vi "FXP_L_ye_Bend_u_singleAxis_32bit.vi"(7 "NS":u8=5, 8 "U(k): ux":fxp<+/-,18,5>, 11 "Y(k): x":fxp<+/-,18,5>) -> (0 "yd_est":fxp<+/-,32,5>, 2 "outputValid":bool, 4 "x0":T1)   [LabVIEW 2017]
uses:
  typeDefs/x_vec_type.ctl
  <vilib>/Platform/TimedLoop/XDataNode/timing_clust.ctl
  <vilib>/Platform/TimedLoop/XDataNode/nitl_modes.ctl
  <vilib>/Platform/TimedLoop/XDataNode/wakeup.ctl
  typeDefs/Lz_bram.ctl
  typeDefs/Bz_bram.ctl
  typeDefs/x_vec_bram.ctl
  <vilib>/rvi/Emulation/niFpgaSctlEmulationGetInTimedLoop.vi
  <vilib>/rvi/Emulation/niFpgaEmulationReportErrorSimple.vi
  <vilib>/rvi/Emulation/niFpgaGetClockAttributes.vi
  <vilib>/rvi/Emulation/niFpgaCriticalErrorInLSC.vi
  <vilib>/rvi/DataTransferAndStorage/Container/Common/niFpgaContainerExecOnDevCompGetState.vi
  <vilib>/rvi/Emulation/niFpgaEmulationIsFPGAContextNoSignature.vi
  <vilib>/rvi/DataTransferAndStorage/Container/Common/niFpgaContainerGetUniqueNameForEmu.vi
  <vilib>/rvi/Emulation/niFpgaProcessEmulError.vi
  <vilib>/rvi/errors/nirviReportUnexpectedCaseInternalError (U32).vi
  <vilib>/rvi/Memory/Memory_Emulation/niFpgaMemoryEmulationCacheClearOnFirstRun.vi
  <vilib>/rvi/Memory/Memory_Emulation/nirvimemoryEmulationManagerCache_MakeExclusive.vi
  <vilib>/rvi/Memory/Memory_Emulation/niFpgaMemoryEmulationValidateCache.vi
  <vilib>/rvi/Memory/Memory_Emulation/nirvimemoryEmulationManagerCache_InsertValue.vi
  <vilib>/Utility/error.llb/Clear Errors.vi
  <vilib>/rvi/Memory/Memory_Emulation/nirvimemoryEmulationManagerCache_ReleaseExclusive.vi
  <vilib>/rvi/Memory/Memory_Emulation/nirvimemoryEmulationManagerCache_GetValue.vi
  <vilib>/rvi/Memory/Memory_Emulation/nirvimemoryEmulationManagerCache_SetValue.vi
  <vilib>/rvi/Emulation/niFpgaSctlEmulationResourceMgr.vi
  <vilib>/Platform/TimedLoop/XDataNode/XDataNode.xnode
  <vilib>/rvi/DataTransferAndStorage/Container/XNode/niFpgaContainer.xnode
  <vilib>/rvi/Memory/Memory_Emulation/niFpgaMemoryEmulationRefIn.vi
  <vilib>/rvi/FXPMathLib/FxpAdd/XNode/nifxpmath_Add.xnode
  <vilib>/Platform/TimedLoop/XDataNode/XDNodeRunTimeDep.lvlib
  <vilib>/rvi/FXPMathLib/sim/FxpSim.dll
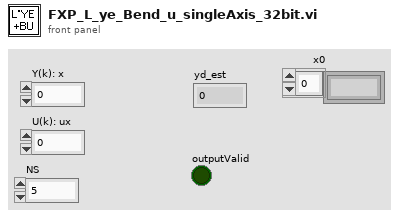
[diagram p1: front panel]
types:
  T1 = typedef "x_vec_type.ctl" = fxp<+/-,32,6>[]
  T2 = typedef "XDNodeRunTimeDep.lvlib/timing_clust.ctl" = cluster{"Expected End [f-1]":u64, "Actual End [f-1]":u64, "Finished Late? [f-1]":bool, "Expected End [i-1]":u64, "Actual End [i-1]":u64, "Finished Late? [i-1]":bool, "Expected Start [i]":u64, "Actual Start [i]":u64, "Expected Start [f]":u64, "Actual Start [f]":u64, "Source Name":string, "Structure Name":string, "Period":i64, "Deadline":i64, "Offset":i64, "Start":i64, "Priority":i32, "Timeout":i32, "Mode":T3, "Wakeup Reason":T4, "Error":errorcluster, "Source Type":string, "Secondary Source Type":string, "Global End Time":u64, "Global Start Time":u64, "Frame Duration":u64, "Iteration Duration":u64, "Assigned CPU":i32, "I/O Scan Engine Mode":u32}
  T3 = typedef "XDNodeRunTimeDep.lvlib/nitl_modes.ctl" = enum32{"No Change", "Process missed periods, maintain original phase", "Discard missed periods, maintain original phase", "Process missed periods, ignore original phase", "Discard missed periods, ignore original phase"}
  T4 = typedef "XDNodeRunTimeDep.lvlib/wakeup.ctl" = enum32{"Normal", "Aborted", "Asynchronous wakeup", "Timing source error", "Timed loop error", "Timeout"}
  T5 = typedef "x_vec_bram.ctl" = refnum<k21>
  T6 = typedef "Bz_bram.ctl" = refnum<k21>
  T7 = typedef "Lz_bram.ctl" = refnum<k21>
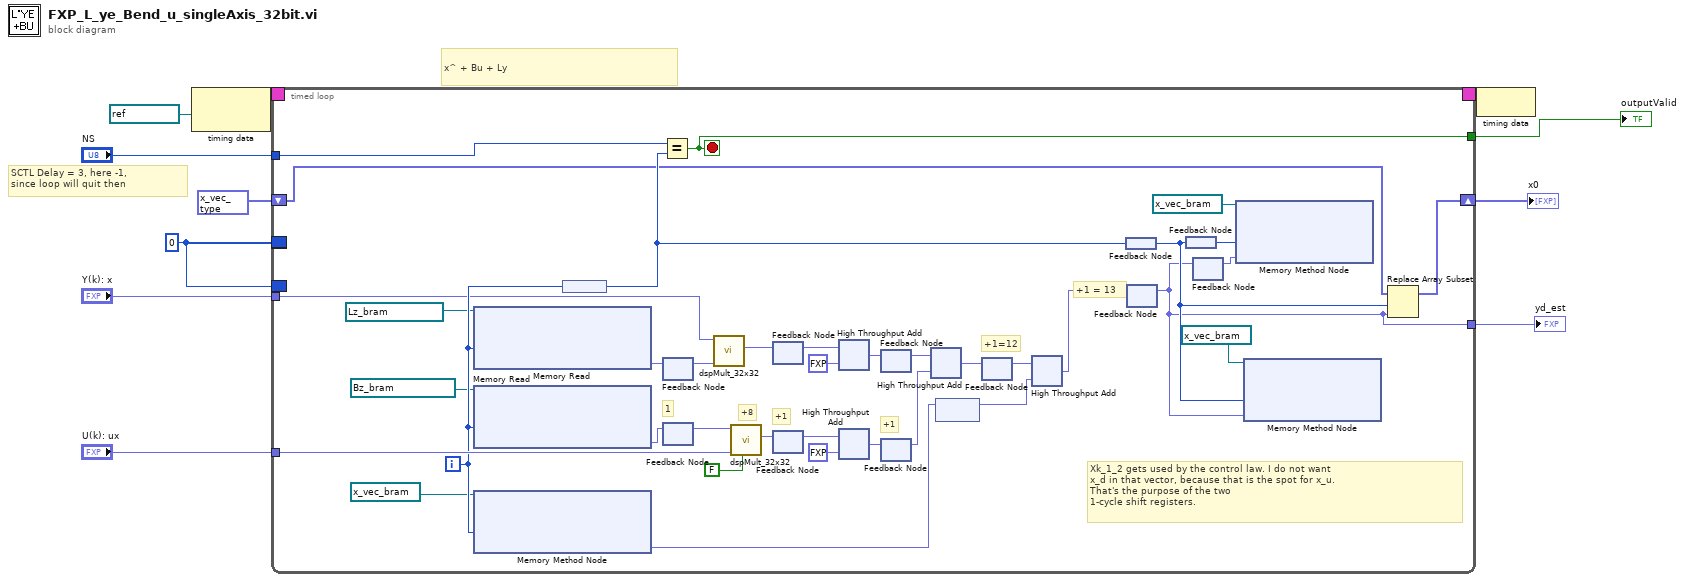
[diagram p0: block diagram]
diagram:
  w6 = 0
  # "x^ + Bu + Ly"
  # "SCTL Delay = 3, here -1,\nsince loop will quit then"
  n1 = node-c288(refnum<k21> "80MHz" ("Source Name")) -> (w11:T2)
  n2 = timed-loop {
    timing: w11 -> [_]
    timing-out: [_] -> w10
    tunnel: "NS" -> [w48]
    border: w6 -> [_]
    tunnel: [w46] -> w8
    border: w6 -> [_]
    tunnel: "Y(k): x" -> [w23]
    tunnel: "U(k): ux" -> [w28]
    border: w6 -> [_]
    tunnel: [w17] -> w5
    shift-right: [w20] -> w2
    shift-left: T1 [0.0, 0.0, 0.0, 0.0, 0.0, 0.0, 0.0, 0.0, 0.0, 0.0, 0.0, 0.0, 0.0, 0.0, 0.0, 0.0, 0.0, 0.0, 0.0, 0.0, 0.0, 0.0, 0.0, 0.0, 0.0] ("Array") -> [w19]
    i -> [w26]
    stop <- w46 stop-if-true
    # "+1 = 13"
    # "+1=12"
    # "+1"
    # "+1"
    # "+8"
    # "1"
    # "Xk_1_2 gets used by the control law. I do not want\nx_d in that vector, because that is the spot for x_u.\nThat's the purpose of the two \n1-cycle shift registers."
    n3 = xnode ("Memory Read")("Address"=w26, "Memory In"=T7 "L_FXP_col1" ("Memory")) -> ("Data"=w44:fxp<+/-,32,3>)  [unwired: 1 out]
    n4 = xnode ("Memory Read")("Address"=w26, "Memory In"=T6 "Bz_FXP_col1" ("Memory")) -> ("Data"=w47:fxp<+/-,32,3>)  [unwired: 1 out]
    n5 = xnode ("Memory Method Node")("Address"=w26, "Memory In"=T5 "xk_1_0" ("Memory")) -> ("Data"=w45:fxp<+/-,32,6>)  [unwired: 1 out]
    n6 = feedback #1() -> (w34:i32)
    n7 = feedback-in #1(w26) -> ()
    n8 = Equal?(x=w48, y=w34) -> (x = y?=w46:bool)
    n9 = feedback #2() -> (w31:fxp<+/-,32,3>)  [unwired: 1 in]
    n10 = feedback-in #2(w44) -> ()
    n11 = feedback #3() -> (w30:fxp<+/-,32,3>)  [unwired: 1 in]
    n12 = feedback-in #3(w47) -> ()
    n13 = call "dspMult_32x32.vi"("b"=w31, "a"=w23) -> ("p"=w32:fxp<+/-,64,10>)  [unwired: 9 in]
    n14 = call "dspMult_32x32.vi"("sclr"=FALSE ("input valid"), "b"=w28, "a"=w30) -> ("p"=w29:fxp<+/-,64,10>)  [unwired: 8 in]
    n15 = feedback #4() -> (w41:fxp<+/-,64,10>)  [unwired: 1 in]
    n16 = feedback-in #4(w32) -> ()
    n17 = feedback #5() -> (w38:fxp<+/-,64,10>)  [unwired: 1 in]
    n18 = feedback-in #5(w29) -> ()
    n19 = xnode ("High Throughput Add")("x"=w41, "y"=fxp<+/-,64,10> 0.0) -> ("x+y"=w40:fxp<+/-,32,8>)
    n20 = xnode ("High Throughput Add")("x"=w38, "y"=fxp<+/-,64,10> 0.0) -> ("x+y"=w37:fxp<+/-,32,8>)
    n21 = feedback #6() -> (w39:fxp<+/-,32,8>)  [unwired: 1 in]
    n22 = feedback-in #6(w40) -> ()
    n23 = feedback #7() -> (w36:fxp<+/-,32,8>)  [unwired: 1 in]
    n24 = feedback-in #7(w37) -> ()
    n25 = xnode ("High Throughput Add")("x"=w39, "y"=w36) -> ("x+y"=w43:fxp<+/-,32,8>)
    n26 = feedback #8() -> (w35:fxp<+/-,32,6>)  [unwired: 1 in]
    n27 = feedback-in #8(w45) -> ()
    n28 = feedback #9() -> (w42:fxp<+/-,32,8>)  [unwired: 1 in]
    n29 = feedback-in #9(w43) -> ()
    n30 = xnode ("High Throughput Add")("x"=w42, "y"=w35) -> ("x+y"=w21:fxp<+/-,32,5>)
    n31 = feedback #10() -> (w18:i32)
    n32 = feedback-in #10(w34) -> ()
    n33 = feedback #11() -> (w17:fxp<+/-,32,5>)  [unwired: 1 in]
    n34 = feedback-in #11(w21) -> ()
    n35 = feedback #12() -> (w22:i32)
    n36 = feedback-in #12(w18) -> ()
    n37 = feedback #13() -> (w33:fxp<+/-,32,5>)  [unwired: 1 in]
    n38 = feedback-in #13(w17) -> ()
    n39 = xnode ("Memory Method Node")("Address"=w22, "Data"=w33, "Memory In"=T5 "xk_1_2" ("Memory")) -> ()  [unwired: 1 out]
    n40 = xnode ("Memory Method Node")("Address"=w18, "Data"=w17, "Memory In"=T5 "xk_1_1" ("Memory")) -> ()  [unwired: 1 out]
    n41 = Replace Array Subset(array=w19, new element=w17, index=w18) -> (w20:T1)
  }
  "outputValid" <- w8
  "yd_est" <- w5
  "x0" <- w2
  n42 = node-c288(w10) -> ()
